vi "2016 Shooter Immediate.vi"(7 "Description":string, 8 "Command Info In":T1, 9 "Deadband Value":dbl=0.01, 11 "Setpoint":dbl) -> (0 "Command Info Out":T1)   [LabVIEW 2016]
uses:
  <vilib>/Rock Robotics/WPI/Framework/Command Status Info.ctl
  <vilib>/Rock Robotics/WPI/Framework/Completion Status.ctl
  <vilib>/Rock Robotics/WPI/Framework/Completion Notifier.ctl
  Implementation/2016 Shooter Setpoints.ctl
  Implementation/2016 Shooter Operations.ctl
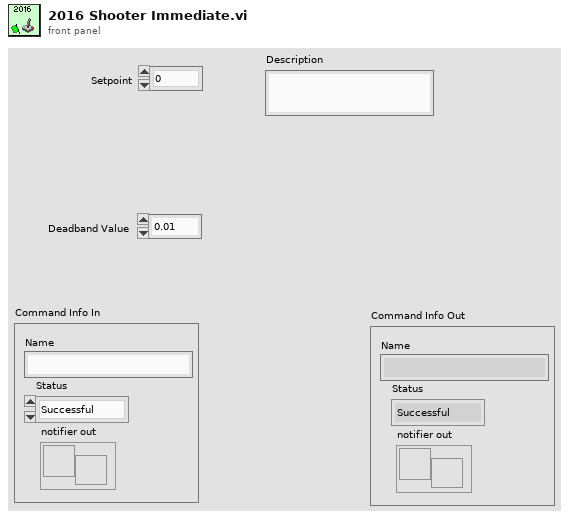
[diagram p1: front panel]
types:
  T1 = typedef "Command Status Info.ctl" = cluster{"Name":string, "Status":T2, "notifier out":T3}
  T2 = typedef "Completion Status.ctl" = enum16{"Successful", "Aborted", "Incomplete"}
  T3 = typedef "Completion Notifier.ctl" = refnum<notifier>
  T4 = typedef "2016 Shooter Setpoints.ctl" = cluster{"Operation":T5, "Setpoint":dbl, "Duration":dbl}
  T5 = typedef "2016 Shooter Operations.ctl" = enum16{"Reserve", "Read Current", "Immediate", "Shoot", "Retrieve"}
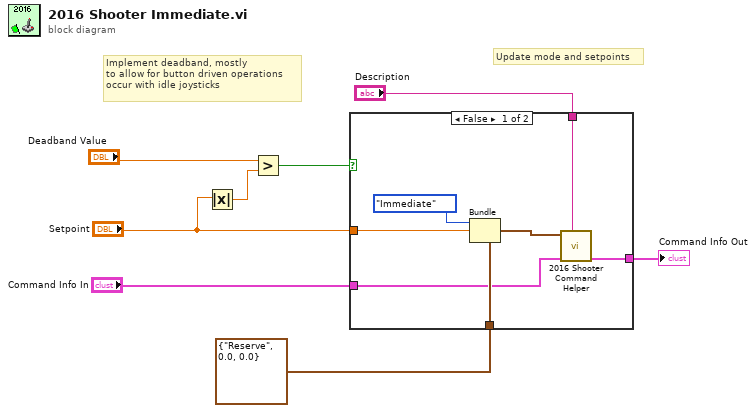
[diagram p0: block diagram]
diagram:
  # "Implement deadband, mostly\nto allow for button driven operations\noccur with idle joysticks"
  # "Update mode and setpoints"
  n1 = Absolute Value(x="Setpoint") -> (abs(x)=w7:dbl)
  n2 = Greater?(x="Deadband Value", y=w7) -> (0:w1:bool)
  n3 = case shown="False" w1 {
    tunnel: "Setpoint" -> [w15 _]
    tunnel: T4 {"Operation"=enum."Reserve", "Setpoint"=0.0, "Duration"=0.0} ("SubSystem Data") -> [w14 _]
    tunnel: [w13 w16] -> w6
    tunnel: "Command Info In" -> [w12 w16]
    tunnel: "Description" -> [w10 _]
    frame False {
      n4 = Bundle(cluster=w14, "Operation"=2016_Shooter_Operations."Immediate", "Setpoint"=w15) -> (w11:T4)  [unwired: 1 in]
      n5 = call "2016 Shooter Command Helper.vi"("Description"=w10, "Command Info In"=w12, "SubSystem Data"=w11) -> ("Command Info Out"=w13:T1)  [unwired: 7 in, 1 out]
    }
    frame True {
    }
  }
  "Command Info Out" <- w6
